vi "Read States.vi"(8 "error in (no error)":errorcluster, 11 "CSM-Helper in":refnum<class "CSM-Helper.lvclass">) -> (0 "error out":errorcluster, 2 "Value":string[](array[string]), 3 "CSM-Helper out":refnum<class "CSM-Helper.lvclass">)   [LabVIEW 2020, in "CSM-Helper.lvclass"]
uses:
  CSM-Helper.lvclass
  CSM-Helper.lvclass/CSM-Helper.ctl
  <userlib>/_NEVSTOP/Communicable State Machine(CSM)/Communicable State Machine.lvlib
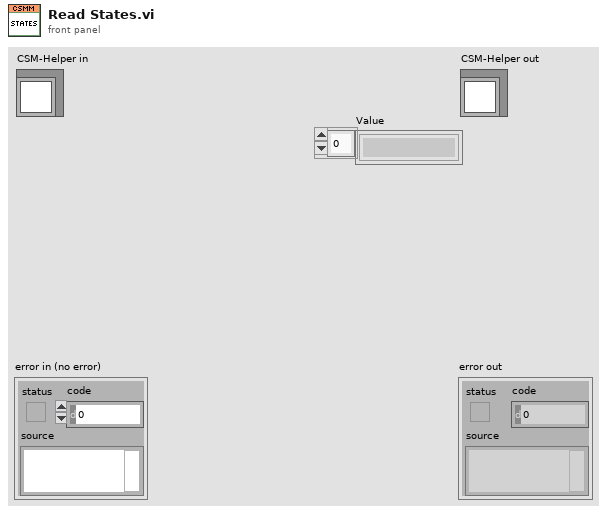
[diagram p1: front panel]
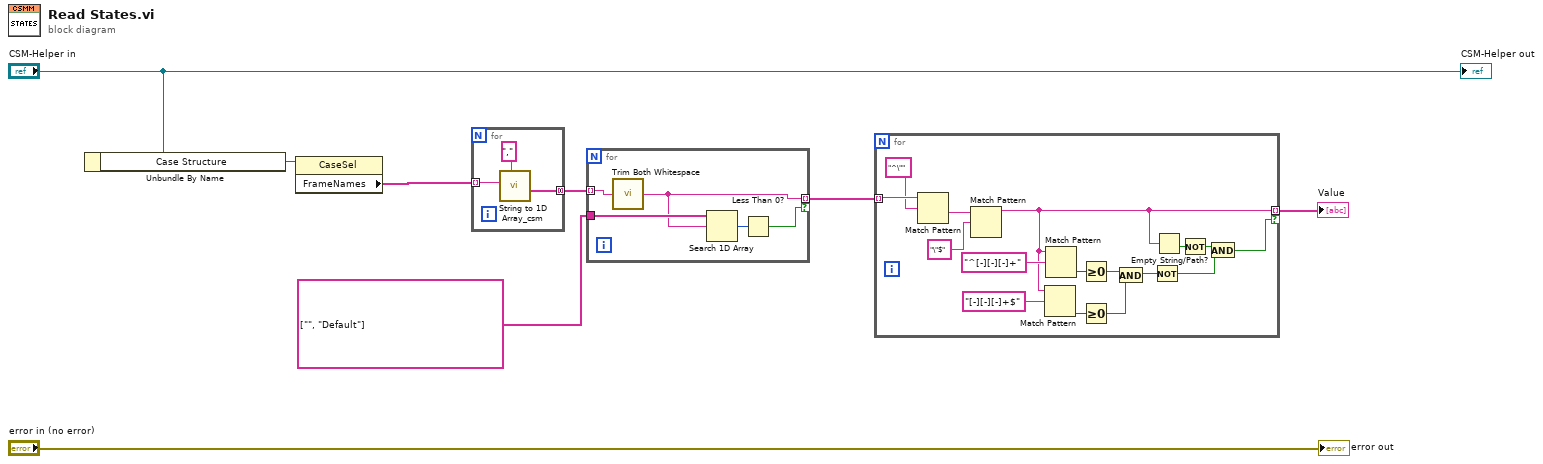
[diagram p0: block diagram]
diagram:
  n1 = Unbundle By Name("CSM-Helper in") -> ("Case Structure"=w4:refnum<vi>)
  n2 = property on="Property Node" class="CaseSel"(reference=w4) -> ("FrameNames"=w8:string[])  [unwired: 1 in, 2 out]
  n3 = for {
    tunnel: w8 -> [w11] mode=indexing
    tunnel: [w9] -> w7 mode=concatenating
    n4 = call <userlib>:"String to 1D Array_csm.vi"("delimiter (Tab)"=",", "string"=w11) -> ("Array of Strings"=w9:string[])  [unwired: 9 in]
  }
  n5 = for {
    tunnel: w7 -> [w16] mode=indexing
    tunnel: [w14] -> w6 mode=indexing if=w12
    tunnel: string[] ["", "Default"] ("items to filter") -> [w15]
    n6 = call <userlib>:"Trim Both Whitespace.vi"("string"=w16) -> ("trimmed string"=w14:string)  [unwired: 1 in]
    n7 = Search 1D Array(1D array=w15, element=w14) -> (index of element=w13:i32)  [unwired: 1 in]
    n8 = Less Than 0?(x=w13) -> (x < 0?=w12:bool)
  }
  n9 = for {
    tunnel: w6 -> [w32] mode=indexing
    tunnel: [w17] -> w2 mode=indexing if=w21
    n10 = Match Pattern(string=w32, regular expression="^\"") -> (after substring=w30:string)  [unwired: 1 in, 3 out]
    n11 = Match Pattern(string=w30, regular expression="\"$") -> (before substring=w17:string)  [unwired: 1 in, 3 out]
    n12 = Match Pattern(string=w17, regular expression="[-][-][-]+$") -> (offset past match=w25:i32)  [unwired: 1 in, 3 out]
    n13 = Match Pattern(string=w17, regular expression="^[-][-][-]+") -> (offset past match=w26:i32)  [unwired: 1 in, 3 out]
    n14 = Greater Or Equal To 0?(x=w26) -> (x >= 0?=w24:bool)
    n15 = Greater Or Equal To 0?(x=w25) -> (x >= 0?=w23:bool)
    n16 = And(x=w24, y=w23) -> (x .and. y?=w22:bool)
    n17 = Not(x=w22) -> (.not. x?=w20:bool)
    n18 = Empty String/Path?(string/path=w17) -> (empty?=w19:bool)
    n19 = Not(x=w19) -> (.not. x?=w18:bool)
    n20 = And(x=w18, y=w20) -> (x .and. y?=w21:bool)
  }
  "Value" <- w2
  "error out" <- "error in (no error)"
  "CSM-Helper out" <- "CSM-Helper in"
